vi "Read Post Meas_.vi"(8 "error in (no error)":errorcluster, 11 "PAE in":refnum<class "PAE.lvclass">) -> (0 "error out":errorcluster, 2 "Post Meas?":bool, 3 "PAE out":refnum<class "PAE.lvclass">)   [LabVIEW 2018, in "SeqAuto Evaluations.lvlib" / "PAE.lvclass"]
uses:
  PAE.lvclass
  PAE.lvclass/PAE.ctl
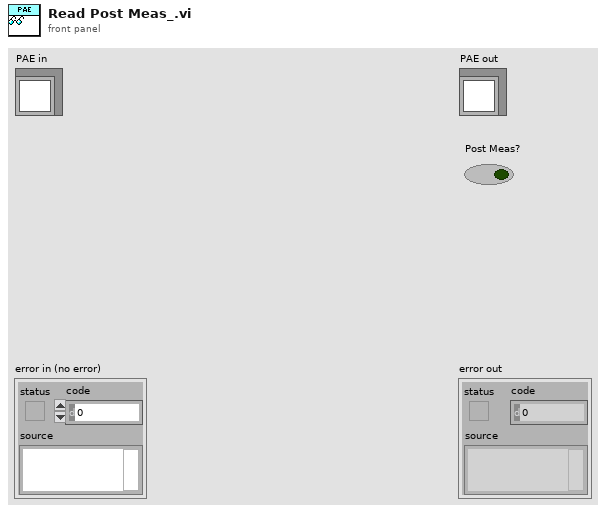
[diagram p1: front panel]
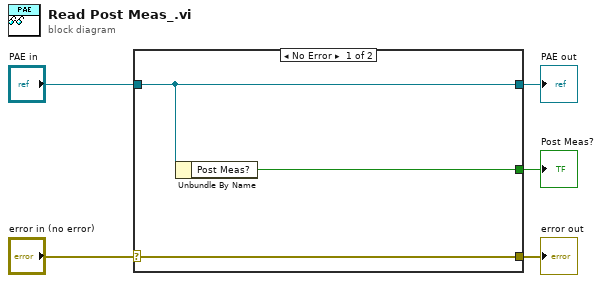
[diagram p0: block diagram]
diagram:
  n1 = case shown="No Error" "error in (no error)" {
    selector: "error in (no error)" -> [w8 w9]
    tunnel: [w8 w9] -> w4
    tunnel: [w7 w10] -> w2
    tunnel: "PAE in" -> [w7 w10]
    tunnel: [w6 _] -> w1
    frame No Error {
      n2 = Unbundle By Name(w7) -> ("Post Meas?"=w6:bool)
    }
    frame Error {
    }
  }
  "error out" <- w4
  "PAE out" <- w2
  "Post Meas?" <- w1
